vi "Turn off Joystick.vi"   [LabVIEW 2015]
doc: "This block is for testing other ESP301 Blocks. Basically it became too annoying to haveto add the connect and disconnect blocks to everything especially if something is not supposed to be a standalone program."
uses:
  <userlib>/Newport ESP301/Newport ESP301.lvlib
panel:
  # "If you run this it will turn the joystick off."
  # "It will also change each axis to s-curve mode. \nI do not know what S-curve mode actually does. \nBut, it allows you to programmatically control \nthe axis motion. When the joystick is turned on \nit sets it to jog mode which will throw alot of \nerrors when youre programming things and trying\n to tell the box what to do and where to go."
types:
  T1 = enum16{"Trapezoidal Mode", "S-curve Mode", "Jog Mode", "Slave to master's desired position (trajectory)", "Slave to master's actual position (feedback)", "Slave to master's actual velocity for jogging"}
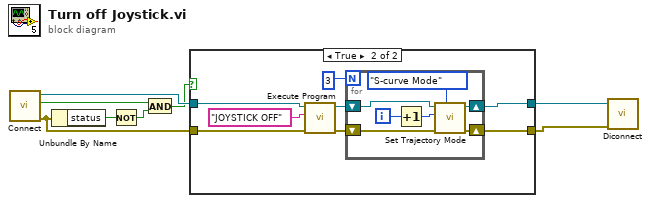
[diagram p0: block diagram]
diagram:
  n1 = call "Connect.vi"() -> ("error out"=w3:errorcluster, "Connected"=w6:bool, "VISA resource name out"=w8:refnum<visa-resource-name>)  [unwired: 5 in]
  n2 = Unbundle By Name(w3) -> ("status"=w7:bool)
  n3 = Not(x=w7) -> (.not. x?=w5:bool)
  n4 = And(x=w6, y=w5) -> (x .and. y?=w4:bool)
  n5 = case shown="True" w4 {
    tunnel: w8 -> [w10 w18]
    tunnel: w3 -> [w9 w17]
    tunnel: [w10 w11] -> w2
    tunnel: [w9 w12] -> w1
    frame False {
    }
    frame True {
      n6 = call <userlib>:"Execute Program.vi"("error in (no error)"=w17, "Program Name"="JOYSTICK OFF", "VISA resource name"=w18) -> ("error out"=w13:errorcluster, "VISA resource name out"=w14:refnum<visa-resource-name>)  [unwired: 3 in]
      n7 = for {
        N: 3 -> [_]
        shift-right: [w20] -> w11
        shift-left: w14 -> [w23]
        shift-right: [w21] -> w12
        shift-left: w13 -> [w22]
        i -> [w25]
        n8 = Increment(x=w25) -> (x+1=w24:i32)
        n9 = call <userlib>:"Set Trajectory Mode.vi"("Trajectory Mode"=T1."S-curve Mode", "error in (no error)"=w22, "Axis (1)"=w24, "VISA resource name"=w23) -> ("error out"=w21:errorcluster, "VISA resource name out"=w20:refnum<visa-resource-name>)  [unwired: 3 in]
      }
    }
  }
  n10 = call "Diconnect.vi"("error in (no error)"=w1, "VISA resource name"=w2) -> ()  [unwired: 6 in]
